vi "Rx Begin.vi"(8 "error in (no error)":errorcluster, 11 "Performance in":refnum<class "Performance.lvclass">) -> (0 "error out":errorcluster, 3 "Performance out":refnum<class "Performance.lvclass">)   [LabVIEW 2017, in "DSF Core.lvlib" / "Performance.lvclass"]
uses:
  Performance.lvclass
  Performance.lvclass/Performance.ctl
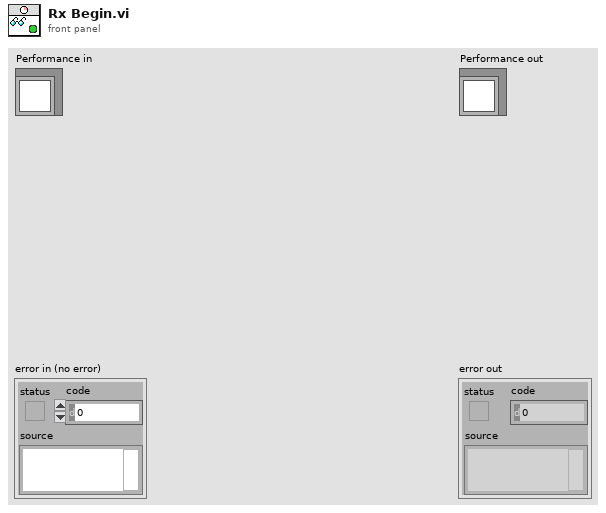
[diagram p1: front panel]
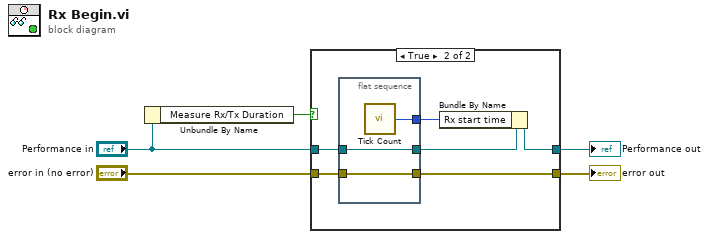
[diagram p0: block diagram]
diagram:
  n1 = Unbundle By Name("Performance in") -> ("Measure Rx/Tx Duration"=w1:bool)
  n2 = case shown="True" w1 {
    tunnel: [w6 w11] -> w5
    tunnel: "error in (no error)" -> [w6 w13]
    tunnel: [w7 w8] -> w3
    tunnel: "Performance in" -> [w7 w12]
    frame False {
    }
    frame True {
      n3 = flat-sequence {
        tunnel: w12 -> [w16]
        tunnel: w13 -> [w15]
        tunnel: [w16] -> w10
        tunnel: [w15] -> w11
        tunnel: [w14] -> w9
        frame #0 {
          n4 = call "Tick Count"() -> ("Tick Count(uSec)"=w14:u32)
        }
      }
      n5 = Bundle By Name(cluster=w10, "Rx start time"=w9) -> (w8:refnum<class "Performance.lvclass">)
    }
  }
  "error out" <- w5
  "Performance out" <- w3
